vi "WPI_CANJaguar_CompareConfig.vi"(4 "Received Data":u8[](array[numeric]), 5 "Expected Data":u8[](array[numeric]), 6 "Message ID":u32) -> (1 "Equivalent":bool)   [LabVIEW 2016]
uses:
  <vilib>/Rock Robotics/WPI/CAN/Jaguar/SubVIs/WPI_CAN_MotorMessageIDs.ctl
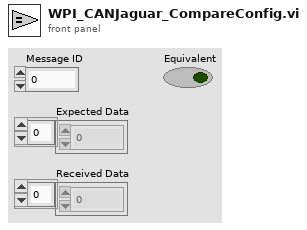
[diagram p1: front panel]
types:
  T1 = typedef "WPI_CAN_MotorMessageIDs.ctl" = u32
  T2 = enum16{"big-endian, network order", "native, host order", "little-endian"}
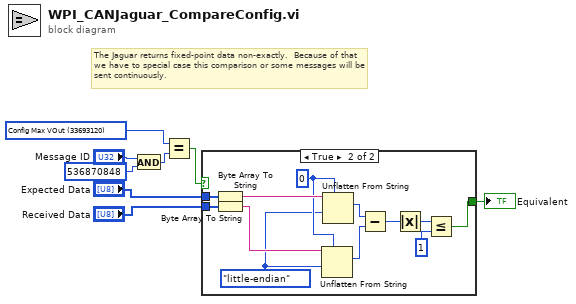
[diagram p0: block diagram]
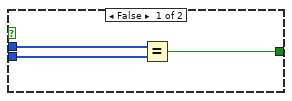
[diagram p2: hidden frame]
diagram:
  w5 = T1 33693120 items=["Volt Enable"=33685504, "Volt Disable"=33685568, "Volt Set"=33685632, "Volt Set Ramp"=33685696, "Speed Enable"=33686528, "Speed Disable"=33686592, "Speed Set"=33686656, "Speed P"=33686720, "Speed I"=33686784, "Speed D"=33686848, "Speed Ref"=33686912, "Volt Comp Enable"=33687552, "Volt Comp Disable"=33687616, "Volt Comp Set"=33687680, "Volt Comp In Ramp"=33687744, "Volt Comp Comp Ramp"=33687808, "Position Enable"=33688576, "Position Disable"=33688640, "Position Set"=33688704, "Position P"=33688768, "Position I"=33688832, "Position D"=33688896, "Position Ref"=33688960, "Current Enable"=33689600, "Current Disable"=33689664, "Current Set"=33689728, "Current P"=33689792, "Current I"=33689856, "Current D"=33689920, "Status Percent VBus"=33690624, "Status VBus"=33690688, "Status Current"=33690752, "Status Temp"=33690816, "Status Position"=33690880, "Status Speed"=33690944, "Status Limit"=33691008, "Status Fault"=33691072, "Status Power"=33691136, "Status Control Mode"=33691200, "Status VOut"=33691264, "Config Num Brushes"=33692672, "Config Encoder Lines"=33692736, "Config Pot Turns"=33692800, "Config Brake Coast"=33692864, "Config Limit Mode"=33692928, "Config Limit Fwd"=33692992, "Config Limit Rev"=33693056, "Config Max VOut"=33693120, "Config Fault Time"=33693184, "Motor Ack"=33693696] ("CAN Motor Message IDs")
  # "The Jaguar returns fixed-point data non-exactly.  Because of that we have to special case this comparison or some messages will be sent continuously."
  n1 = And(x="Message ID", y=u32 536870848) -> (x .and. y?=w1:u32)
  n2 = Equal?(x=w5, y=w1) -> (x = y?=w4:bool)
  n3 = case shown="True" w4 {
    tunnel: "Expected Data" -> [w11 w22]
    tunnel: [w10 w13] -> w7
    tunnel: "Received Data" -> [w9 w23]
    frame False {
      n4 = Equal?(x=w11, y=w9) -> (x = y?=w10:bool)
    }
    frame True {
      w12 = T2."little-endian" ("byte order (0:big-endian, network order)")
      w19 = i16 0
      n5 = Byte Array To String(unsigned byte array=w22) -> (string=w21:string)
      n6 = Byte Array To String(unsigned byte array=w23) -> (string=w20:string)
      n7 = Unflatten From String(type=w19, binary string=w20, byte order (0:big-endian, network order)=w12) -> (value=w17:i16)  [unwired: 2 in, 2 out]
      n8 = Unflatten From String(type=w19, binary string=w21, byte order (0:big-endian, network order)=w12) -> (value=w18:i16)  [unwired: 2 in, 2 out]
      n9 = Subtract(x=w18, y=w17) -> (x-y=w16:i16)
      n10 = Absolute Value(x=w16) -> (abs(x)=w15:i16)
      n11 = Less Or Equal?(x=w15, y=i16 1) -> (x <= y?=w13:bool)
    }
  }
  "Equivalent" <- w7
